vi "N4_201_StandartRangeSelect (SubVI).vi"(0 "RangeCommand":string[](array[string]), 1 "ScaleArray":dbl[](array[numeric]), 2 "RangeDigit":dbl[](array[numeric]), 3 "Control Point":dbl, 5 "error in":errorcluster, 6 "RangeAuto":bool=TRUE, 8 "Range":dbl, 9 "Error Code":i32, 11 "Driver Name":string) -> (14 "R/O":string, 15 "ScaledValue":dbl=1.0, 19 "error out":errorcluster)   [LabVIEW 2018]
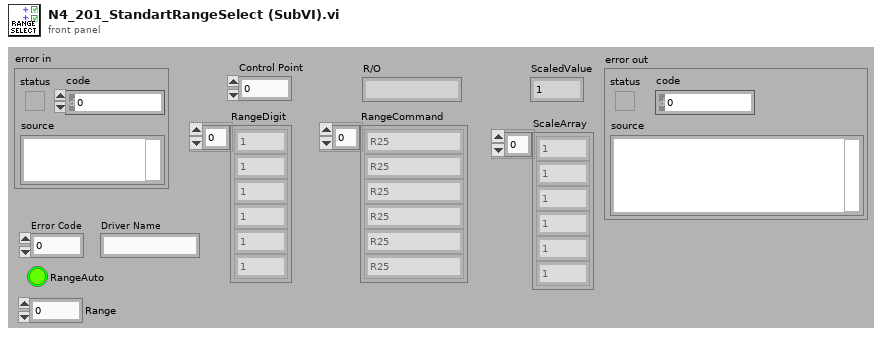
[diagram p1: front panel]
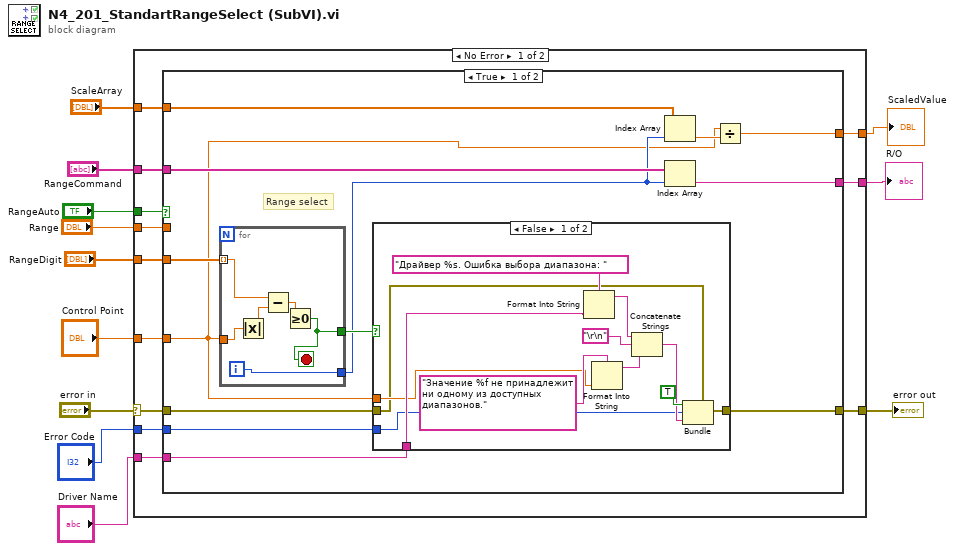
[diagram p0: block diagram]
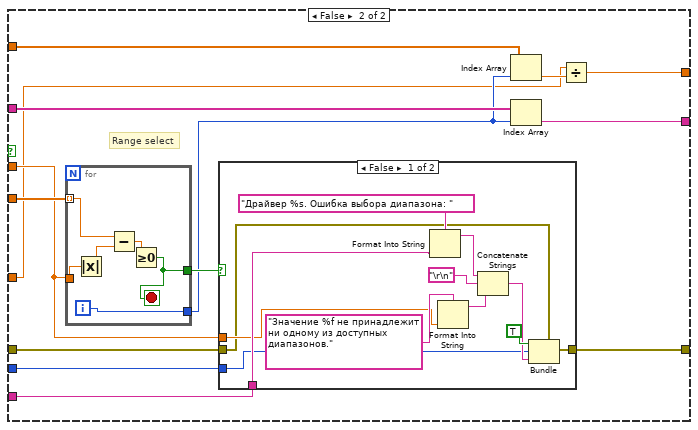
[diagram p3: hidden frame]
diagram:
  n1 = case shown="No Error" "error in" {
    selector: "error in" -> [w21 w90]
    tunnel: "Control Point" -> [w16 _]
    tunnel: "RangeDigit" -> [w24 _]
    tunnel: "RangeCommand" -> [w23 _]
    tunnel: [w18 w90] -> w8
    tunnel: [w22 _] -> w7
    tunnel: "Error Code" -> [w19 _]
    tunnel: "Driver Name" -> [w20 _]
    tunnel: "ScaleArray" -> [w17 _]
    tunnel: [w15 _] -> w3
    tunnel: "RangeAuto" -> [w14 _]
    tunnel: "Range" -> [w13 _]
    frame No Error {
      n2 = case shown="True" w14 {
        tunnel: w24 -> [w37 w70]
        tunnel: w23 -> [w36 w69]
        tunnel: [w34 w67] -> w22
        tunnel: w21 -> [w33 w66]
        tunnel: w20 -> [w32 w65]
        tunnel: w19 -> [w31 w64]
        tunnel: [w30 w63] -> w18
        tunnel: w17 -> [w29 w62]
        tunnel: w16 -> [w26 w57]
        tunnel: [w25 w59] -> w15
        tunnel: w13 -> [_ w58]
        frame True {
          # "Range select"
          n3 = for {
            tunnel: w37 -> [w56] mode=indexing
            tunnel: w26 -> [w55]
            tunnel: [w52] -> w28
            tunnel: [w51] -> w35
            i -> [w52]
            stop <- w51 stop-if-true
            n4 = Absolute Value(x=w55) -> (abs(x)=w54:dbl)
            n5 = Subtract(x=w56, y=w54) -> (x-y=w53:dbl)
            n6 = Greater Or Equal To 0?(x=w53) -> (x >= 0?=w51:bool)
          }
          n7 = case shown="False" w35 {
            tunnel: w33 -> [w39 w50]
            tunnel: w32 -> [w44 _]
            tunnel: w31 -> [w38 _]
            tunnel: w26 -> [w42 _]
            tunnel: [w40 w50] -> w30
            frame False {
              n8 = Format Into String(format string="Драйвер %s. Ошибка выбора диапазона: ", w44) -> (resulting string=w47:string)  [unwired: 2 in, 1 out]
              n9 = Format Into String(format string="Значение %f не принадлежит ни одному из доступных диапазонов." ("string"), w42) -> (resulting string=w41:string)  [unwired: 2 in, 1 out]
              n10 = Concatenate Strings(w47, "\r\n", w41) -> (w45:string)
              n11 = Bundle(cluster=w39, "status"=TRUE ("Status"), "code"=w38, "source"=w45) -> (w40:errorcluster)
            }
            frame True {
            }
          }
          n12 = Index Array(array=w29, index=w28) -> (element=w27:dbl)
          n13 = Index Array(array=w36, index=w28) -> (element=w34:string)
          n14 = Divide(x=w26, y=w27) -> (x/y=w25:dbl)
        }
        frame False {
          # "Range select"
          n15 = for {
            tunnel: w70 -> [w89] mode=indexing
            tunnel: w58 -> [w88]
            tunnel: [w85] -> w61
            tunnel: [w84] -> w68
            i -> [w85]
            stop <- w84 stop-if-true
            n16 = Absolute Value(x=w88) -> (abs(x)=w87:dbl)
            n17 = Subtract(x=w89, y=w87) -> (x-y=w86:dbl)
            n18 = Greater Or Equal To 0?(x=w86) -> (x >= 0?=w84:bool)
          }
          n19 = case shown="False" w68 {
            tunnel: w66 -> [w72 w83]
            tunnel: w65 -> [w77 _]
            tunnel: w64 -> [w71 _]
            tunnel: w58 -> [w75 _]
            tunnel: [w73 w83] -> w63
            frame False {
              n20 = Format Into String(format string="Драйвер %s. Ошибка выбора диапазона: ", w77) -> (resulting string=w80:string)  [unwired: 2 in, 1 out]
              n21 = Format Into String(format string="Значение %f не принадлежит ни одному из доступных диапазонов." ("string"), w75) -> (resulting string=w74:string)  [unwired: 2 in, 1 out]
              n22 = Concatenate Strings(w80, "\r\n", w74) -> (w78:string)
              n23 = Bundle(cluster=w72, "status"=TRUE ("Status"), "code"=w71, "source"=w78) -> (w73:errorcluster)
            }
            frame True {
            }
          }
          n24 = Index Array(array=w62, index=w61) -> (element=w60:dbl)
          n25 = Index Array(array=w69, index=w61) -> (element=w67:string)
          n26 = Divide(x=w57, y=w60) -> (x/y=w59:dbl)
        }
      }
    }
    frame Error {
    }
  }
  "error out" <- w8
  "R/O" <- w7
  "ScaledValue" <- w3
